vi "OutputLED.vi"   [LabVIEW 2020]
doc: "This VI sends commands to the robot LEDs."
uses:
  robotoutputs.vi
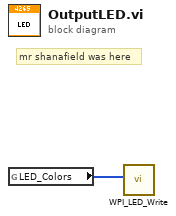
[diagram p0: block diagram]
diagram:
  # "mr shanafield was here"
  n1 = global read "robotoutputs.vi" "LED_Colors"() -> (w1:u32[])
  n2 = call <vilib>:"WPI_LED_Write.vi"("Color Array"=w1) -> ()  [unwired: 10 in, 1 out]
